vi "Std_Bus_Write.vi"(0 "ILabVIEW In":refnum<k24>, 1 "deviceType":i32(ring) items=["Controller", "RUI", "PC", "CommsCard"], 2 "Zone":i32, 3 "ParameterID":i32, 4 "InstanceId":i32, 5 "error in (no error)":errorcluster, 6 "TemperatureUnits":u8(ring) items=["Degrees F", "Degrees C"], 7 "WriteValue":string) -> (14 "ILabVIEW Out":refnum<k24>, 19 "error out":errorcluster)   [LabVIEW 2018]
doc: "This VI is used to Write a parameter specified by the user. Refer to users manual (CIP) Class Instance Attribute column for <B>Parameter ID</B> values.\n\n<B>DeviceType</B> is the type of device being connected to. \nThe selections are:\n <B>Control</B> - This will be from one of the following Watlow controllers (PM Family, RM Family, ST Family and F4T)\n<B> RUI</B> - This will be any Watlow Remote User Interface\n<B> PC</B> - Not used at this time\n<B> CommsCard</B> Not used at this time\n\n<B>Zone</B> is the logical address. Range 1-17.\n\nThe <B>Instance</B> defines the occurrence of the feature.\nExample:\nInput 1 - <B>Instance 1</B>\nInput 2 - <B>Instance 2</B>\nAlarm 1 - <B>Instance 1</B>\nAlarm 2 - <B>Instance 2</B>\nOutput 1 - <B>Instance 1</B>\nOutput 2 - <B>Instance 2</B>\nDIO1 (Output 5) - <B>Instance 5</B>\nDIO2 (Output 6) - <B>Instance 6</B>\netc."
uses:
  C:/RageATE/Instruments/Ess Temp Plate/LabView Driver/Public/Watbus.dll
  Watbus.dll
panel:
  # "Std Bus Write"
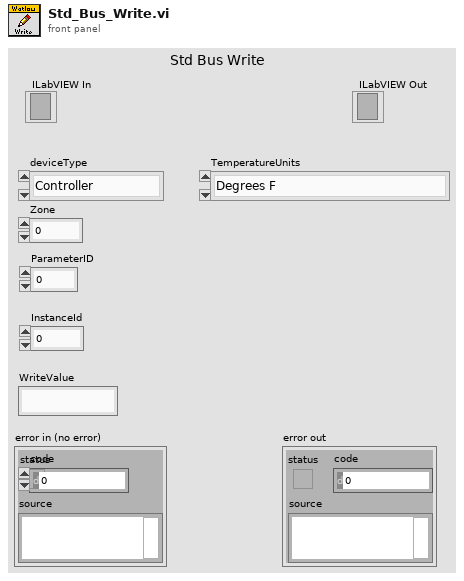
[diagram p1: front panel]
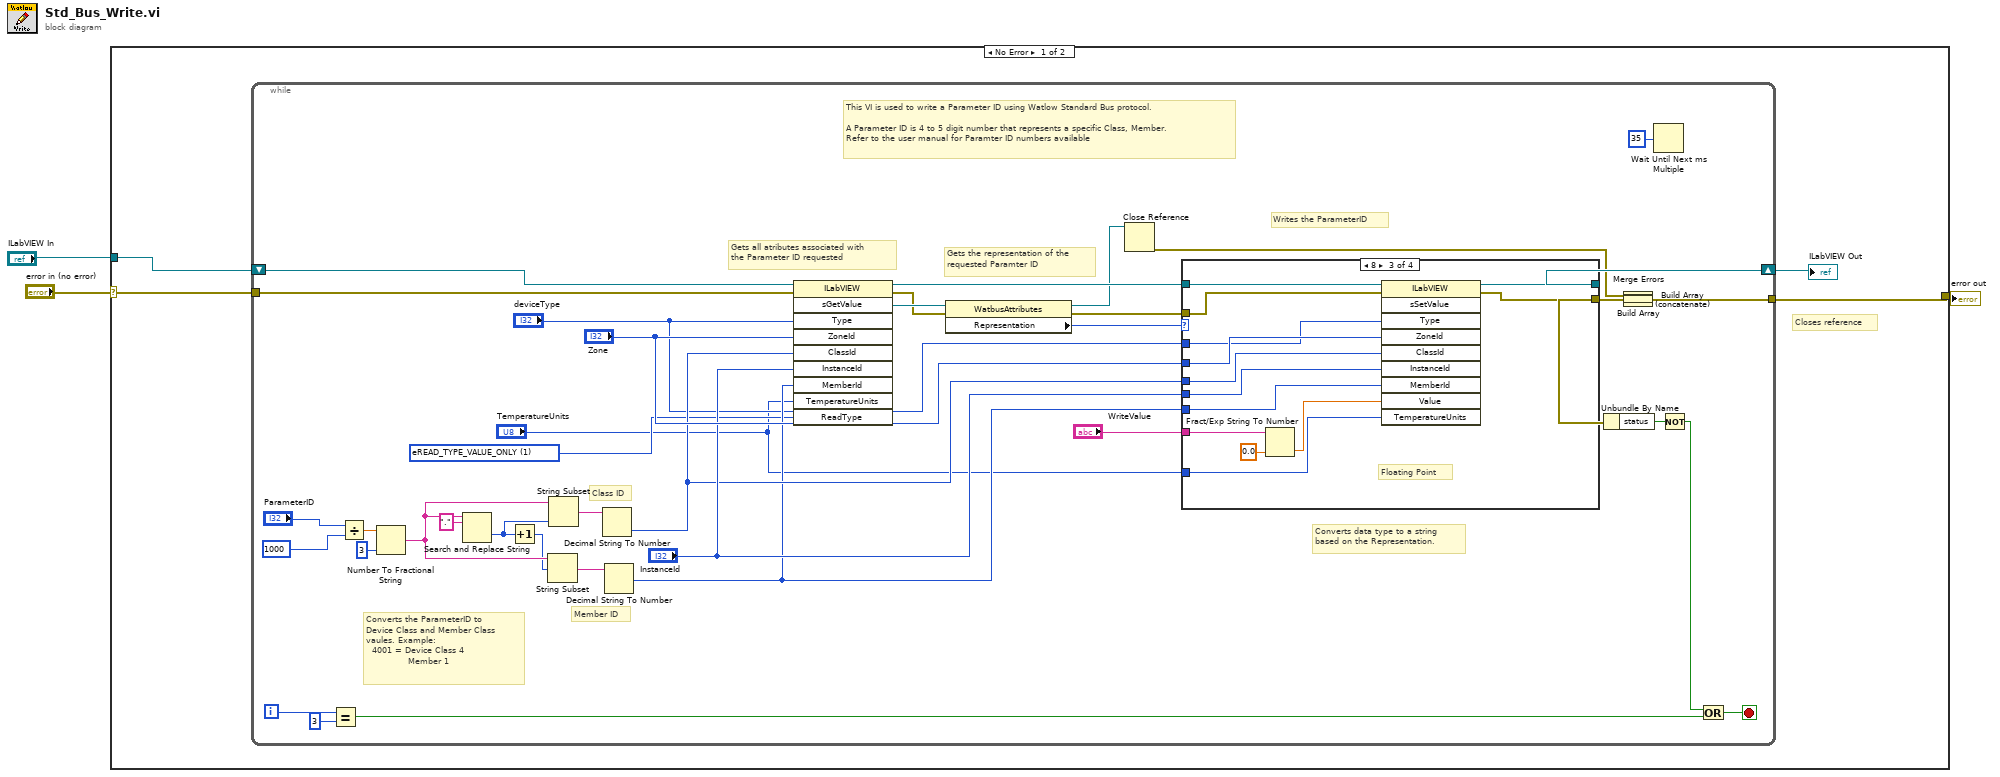
[diagram p0: block diagram]
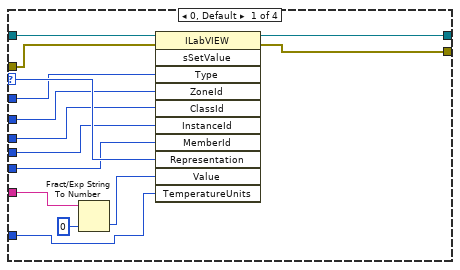
[diagram p2: hidden frame]
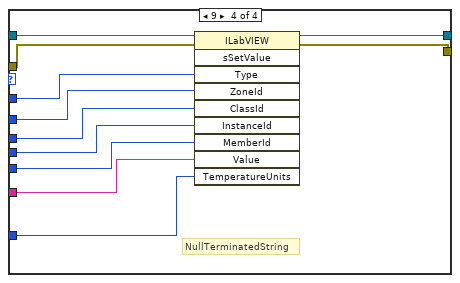
[diagram p4: hidden frame]
diagram:
  n1 = case shown="No Error" "error in (no error)" {
    selector: "error in (no error)" -> [w7 w87]
    tunnel: [w6 w87] -> w3
    tunnel: "ILabVIEW In" -> [w5 _]
    frame No Error {
      # "Closes reference"
      n2 = while {
        tunnel: w7 -> [w46]
        tunnel: [w12] -> w6
        shift-right: [w16] -> w4
        shift-left: w5 -> [w17]
        i -> [w24]
        stop <- w19 stop-if-true
        w10 = u8 1 items=["eREAD_TYPE_VALUE_ONLY"=1, "eREAD_TYPE_VALUE_AND_ATTRIBUTES"=2] ("ReadType")
        # "This VI is used to write a Parameter ID using Watlow Standard Bus protocol.\n\nA Parameter ID is 4 to 5 digit number that represents a specific Class, Member.\nRefer to the user manual for Paramter ID numbers available"
        # "Gets the representation of the\nrequested Paramter ID"
        # "Gets all atributes associated with \nthe Parameter ID requested"
        # "Writes the ParameterID"
        # "Converts data type to a string \nbased on the Representation."
        # "Converts the ParameterID to\nDevice Class and Member Class\nvaules. Example:\n  4001 = Device Class 4\n              Member 1"
        # "Class ID"
        # "Member ID"
        n3 = Equal?(x=w24, y=3) -> (x = y?=w20:bool)
        n4 = Divide(x="ParameterID", y=1000) -> (x/y=w30:dbl)
        n5 = Number To Fractional String(number=w30, precision (6)=i16 3) -> (F-format string=w35:string)  [unwired: 2 out]
        n6 = Search and Replace String(input string=w35, search string=".") -> (offset past replacement=w36:i32)  [unwired: 1 in, 8 out]
        n7 = Increment(x=w36) -> (x+1=w33:i32)
        n8 = String Subset(string=w35, offset (0)=w33) -> (substring=w34:string)  [unwired: 1 out]
        n9 = String Subset(string=w35, length (rest)=w36) -> (substring=w37:string)  [unwired: 1 out]
        n10 = Decimal String To Number(string=w37) -> (number=w27:i32)  [unwired: 3 out]
        n11 = Decimal String To Number(string=w34) -> (number=w26:i32)  [unwired: 3 out]
        n12 = invoke class="ILabVIEW" method="sGetValue"(reference=w17, error in=w46, "Type"="deviceType", "ZoneId"="Zone", "ClassId"=w27, "InstanceId"="InstanceId", "MemberId"=w26, "TemperatureUnits"="TemperatureUnits", "ReadType"=w10) -> (reference out=w42:refnum<k24>, error out=w44:errorcluster, "sGetValue"=w45:refnum<k24>)  [unwired: 1 in, 7 out]
        n13 = property class="WatbusAttributes"(reference=w45, error in=w44) -> (reference out=w15:refnum<k24>, error out=w40:errorcluster, "Representation"=w43:i32)
        n14 = Close Reference(reference=w15) -> (error out=w14:errorcluster)  [unwired: 1 in]
        n15 = case shown="8" w43 {
          selector: w43 -> [w54 _ _ _]
          tunnel: w42 -> [w60 w62 w73 w86]
          tunnel: "WriteValue" -> [w59 _ w75 w77]
          tunnel: w40 -> [w57 w61 w72 w83]
          tunnel: [w56 w62 w71 w85] -> w16
          tunnel: [w55 w61 w70 w84] -> w13
          tunnel: "Zone" -> [w52 _ w66 w79]
          tunnel: w27 -> [w51 _ w67 w80]
          tunnel: "InstanceId" -> [w50 _ w68 w81]
          tunnel: w26 -> [w49 _ w69 w82]
          tunnel: "deviceType" -> [w53 _ w65 w78]
          tunnel: "TemperatureUnits" -> [w47 _ w63 w76]
          frame 0, Default {
            n16 = Fract/Exp String To Number(string=w59, default (0 dbl)=i64 0 ("default (0 DBL)")) -> (number=w48:i64)  [unwired: 3 out]
            n17 = invoke class="ILabVIEW" method="sSetValue"(reference=w60, error in=w57, "Type"=w53, "ZoneId"=w52, "ClassId"=w51, "InstanceId"=w50, "MemberId"=w49, "Representation"=w54, "Value"=w48, "TemperatureUnits"=w47) -> (reference out=w56:refnum<k24>, error out=w55:errorcluster)  [unwired: 1 in, 9 out]
          }
          frame 7, 10 {
            # "Writing to a list is not supported at this time"
            # "EnumertatedList\nListOfBits"
          }
          frame 8 {
            # "Floating Point"
            n18 = Fract/Exp String To Number(string=w75, default (0 dbl)=sgl 0.0 ("default (0 DBL)")) -> (number=w64:sgl)  [unwired: 3 out]
            n19 = invoke class="ILabVIEW" method="sSetValue"(reference=w73, error in=w72, "Type"=w65, "ZoneId"=w66, "ClassId"=w67, "InstanceId"=w68, "MemberId"=w69, "Value"=w64, "TemperatureUnits"=w63) -> (reference out=w71:refnum<k24>, error out=w70:errorcluster)  [unwired: 1 in, 8 out]
          }
          frame 9 {
            # "NullTerminatedString"
            n20 = invoke class="ILabVIEW" method="sSetValue"(reference=w86, error in=w83, "Type"=w78, "ZoneId"=w79, "ClassId"=w80, "InstanceId"=w81, "MemberId"=w82, "Value"=w77, "TemperatureUnits"=w76) -> (reference out=w85:refnum<k24>, error out=w84:errorcluster)  [unwired: 1 in, 8 out]
          }
        }
        n21 = Unbundle By Name(w13) -> ("status"=w22:bool)
        n22 = Build Array(w14, w13) -> (w11:errorcluster[])
        n23 = Build Array (concatenate)(w11) -> (w8:errorcluster[])
        n24 = Merge Errors(w8) -> (w12:errorcluster)
        n25 = Wait Until Next ms Multiple(millisecond multiple=u32 35) -> ()  [unwired: 1 out]
        n26 = Not(x=w22) -> (.not. x?=w21:bool)
        n27 = Or(x=w21, y=w20) -> (x .or. y?=w19:bool)
      }
      "ILabVIEW Out" <- w4
    }
    frame Error {
    }
  }
  "error out" <- w3
